vi "set source.vi"(10 "source":string, 11 "exception in":T1 {"code" format="%.0x"}) -> (3 "exception out":T1 {"code" format="%.0x"})   [LabVIEW 2013, in "exception.lvlib"]
uses:
  exception.lvlib
  exception.ctl
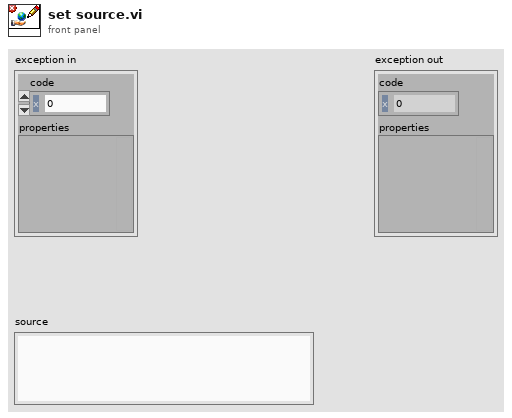
[diagram p1: front panel]
types:
  T1 = typedef "exception.lvlib/exception.ctl" = cluster{"code":i32, "properties":variant}
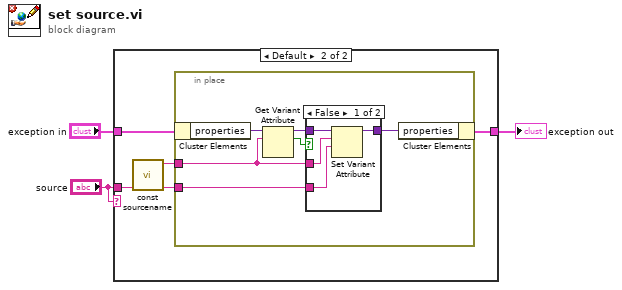
[diagram p0: block diagram]
diagram:
  n1 = case shown="Default" "source" {
    tunnel: "exception in" -> [w4 w8]
    tunnel: [w4 w7] -> w2
    tunnel: "source" -> [_ w5]
    frame "" {
    }
    frame Default {
      n2 = call "const sourcename.vi"() -> ("label"=w6:string)  [unwired: 11 in]
      n3 = in-place {
        in-place-border: w6 -> [w10]
        in-place-border: w5 -> [w13]
        n4 = in-place-cluster #1(w8) -> ("properties"=w11:variant)
        n5 = Get Variant Attribute(Variant=w11, name=w10) -> (duplicate Variant=w12:variant, found=w9:bool)  [unwired: 2 in, 2 out]
        n6 = case shown="False" w9 {
          tunnel: [w18 w19] -> w14
          tunnel: w13 -> [w17 _]
          tunnel: w12 -> [w16 w19]
          tunnel: w10 -> [w15 _]
          frame False {
            n7 = Set Variant Attribute(Variant=w16, name=w15, value=w17) -> (Variant out=w18:variant)  [unwired: 1 in, 2 out]
          }
          frame True {
          }
        }
        n8 = in-place-cluster #1("properties"=w14) -> (w7:T1)
      }
    }
  }
  "exception out" <- w2
